vi "Convert SN bytes to SN data.vi"(11 "SN Data Bytes":u8[](array[numeric]) format="%.0x") -> (2 "SN":string, 3 "SN":u32)   [LabVIEW 2025]
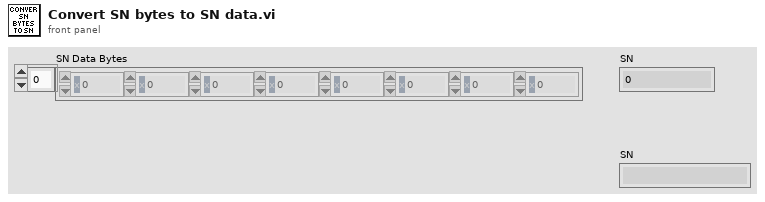
[diagram p1: front panel]
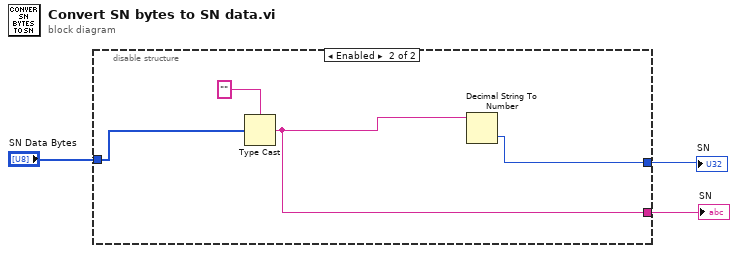
[diagram p0: block diagram]
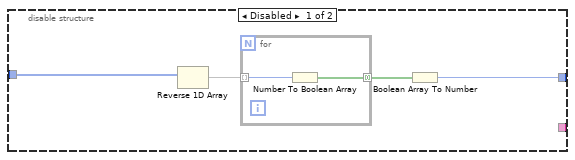
[diagram p2: hidden frame]
diagram:
  n1 = disable-structure shown="Enabled" {
    disable-tunnel: "SN Data Bytes" -> [w5 w12]
    disable-tunnel: [w4 w11] -> w2
    disable-tunnel: [_ w10] -> w1
    frame Disabled {
      n2 = Reverse 1D Array(array=w5) -> (reversed array=w7:u8[])
      n3 = for {
        tunnel: w7 -> [w9] mode=indexing
        tunnel: [w8] -> w6 mode=concatenating
        n4 = Number To Boolean Array(number=w9) -> (Boolean array=w8:bool[])
      }
      n5 = Boolean Array To Number(Boolean array=w6) -> (number=w4:u32)
    }
    frame Enabled {
      n6 = Type Cast(type="" ("HW part number"), x=w12) -> (*(type *) &x=w10:string)
      n7 = Decimal String To Number(string=w10) -> (number=w11:i32)  [unwired: 2 in, 1 out]
    }
  }
  "SN" <- w2
  "SN" <- w1
